vi "Shooter_WinchNoPID.vi"(8 "Winch Pot Location":dbl, 10 "selectedCase":i32, 11 "SetPointArray":dbl[](array[numeric])=[1.0, 2.0, 3.0]) -> (3 "Winch Motor Power Out":dbl)   [LabVIEW 2013]
panel:
  in  "WinchPower":dbl=0.75
  out "Winch Desired Location":dbl
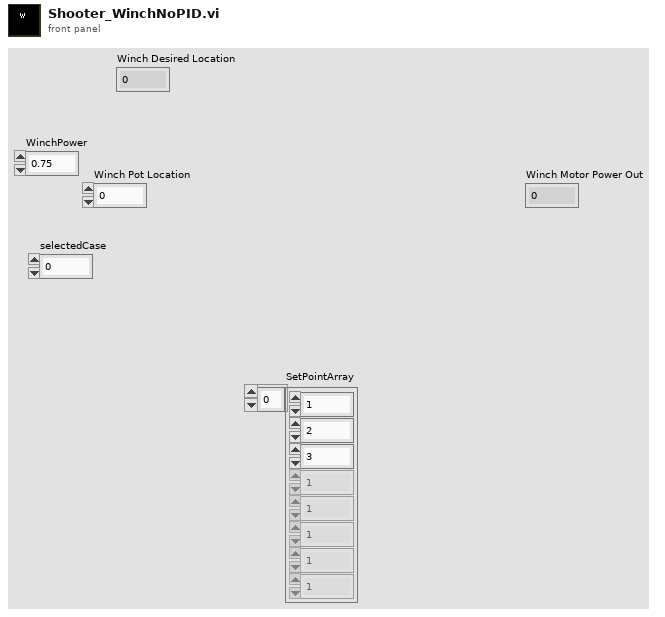
[diagram p1: front panel]
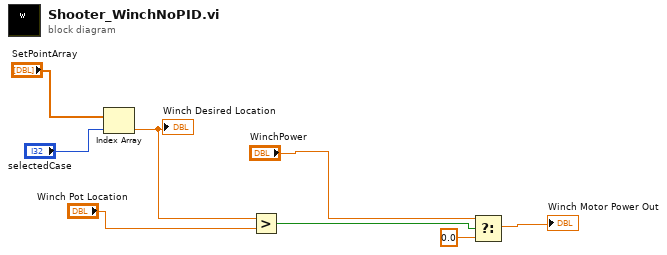
[diagram p0: block diagram]
diagram:
  n1 = Index Array(array="SetPointArray", index="selectedCase") -> (element=w3:dbl)
  "Winch Desired Location" <- w3
  n2 = Greater?(x=w3, y="Winch Pot Location") -> (0:w1:bool)
  n3 = Select(t="WinchPower", s=w1, f=0.0) -> (s? t:f=→"Winch Motor Power Out":dbl)
